vi "test Verify Timestamp Channels Created.vi"(8 "error in":errorcluster, 11 "TestCase in":refnum<class "Scripting.lvclass">) -> (0 "error out":errorcluster, 3 "TestCase out":refnum<class "Scripting.lvclass">)   [LabVIEW 2020, in "Scripting.lvclass"]
uses:
  Scripting.lvclass
  C:/dev/git/niveristand-custom-device-testing-tools/VeriStandScriptingTestCase/VeriStandScriptingTestCase.lvclass
  Shared/BIU Configuration.ctl
  Shared/Address.ctl
  Shared/Major Frame Definition.ctl
  Shared/Minor Frame Definition.ctl
  Shared/Acyclic Frame Definition.ctl
  Shared/Message Definition.ctl
  Shared/Message Type.ctl
  Shared/Terminal Endpoint.ctl
  Shared/Parameter Definition.ctl
  niveristand-custom-device-testing-tools/VeriStandScriptingTestCase/VeriStandScriptingTestCase.lvclass/VeriStandScriptingTestCase.ctl
  niveristand-custom-device-testing-tools/VeriStandScriptingTestCase/Read Target.vi
  Scripting/Constants.vi
  <vilib>/NI VeriStand/Custom Device Tools/Custom Device Utility Library/NI VeriStand - Search for All Items by GUID.vi
  NationalInstruments.VeriStand.SystemDefinitionAPI
  <vilib>/addons/_JKI Toolkits/VI Tester/TestCase.llb/TestCase.lvclass
  Scripting/AIM MIL-STD-1553 Scripting.lvlib
  <vilib>/NI VeriStand/Custom Device Tools/Custom Device Utility Library/Custom Device Utility Library.lvlib
  C:/Program Files (x86)/National Instruments/LabVIEW 2020/vi.lib/addons/_JKI Toolkits/VI Tester/TestCase.llb/TestCase.lvclass
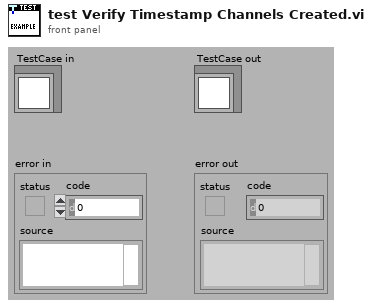
[diagram p1: front panel]
types:
  T1 = typedef "BIU Configuration.ctl" = cluster{"HW channel":u16, "terminal addresses":T2[], "terminal names":string[], "major frames":T3[], "minor frames":T4[], "acyclic frames":T5[], "messages":T6[], "minor frame period (us)":i32}
  T2 = typedef "Address.ctl" = u16
  T3 = typedef "Major Frame Definition.ctl" = cluster{"name":string, "minor frames":string[]}
  T4 = typedef "Minor Frame Definition.ctl" = cluster{"name":string, "messages":string[]}
  T5 = typedef "Acyclic Frame Definition.ctl" = cluster{"name":string, "messages":string[]}
  T6 = typedef "Message Definition.ctl" = cluster{"name":string, "message type":T7, "endpoint Tx":T8, "endpoint Rx":T8, "create timestamp channel":bool, "mode code":u16, "number of words":u16, "parameters":cluster{"name":string, "default value":dbl, "unit":string, "parameter definition":T9}[]}
  T7 = typedef "Message Type.ctl" = string
  T8 = typedef "Terminal Endpoint.ctl" = cluster{"terminal address":T2, "subaddress":T2}
  T9 = typedef "Parameter Definition.ctl" = cluster{"start index":i32, "size (bits)":i32, "encoding":enum16{"BNR", "BCD", "Discrete"}, "signed":bool, "multiplier":dbl, "offset":dbl}
  T10 = typedef "Custom Device API.lvlib/Custom Device Item Ref.ctl" = u64
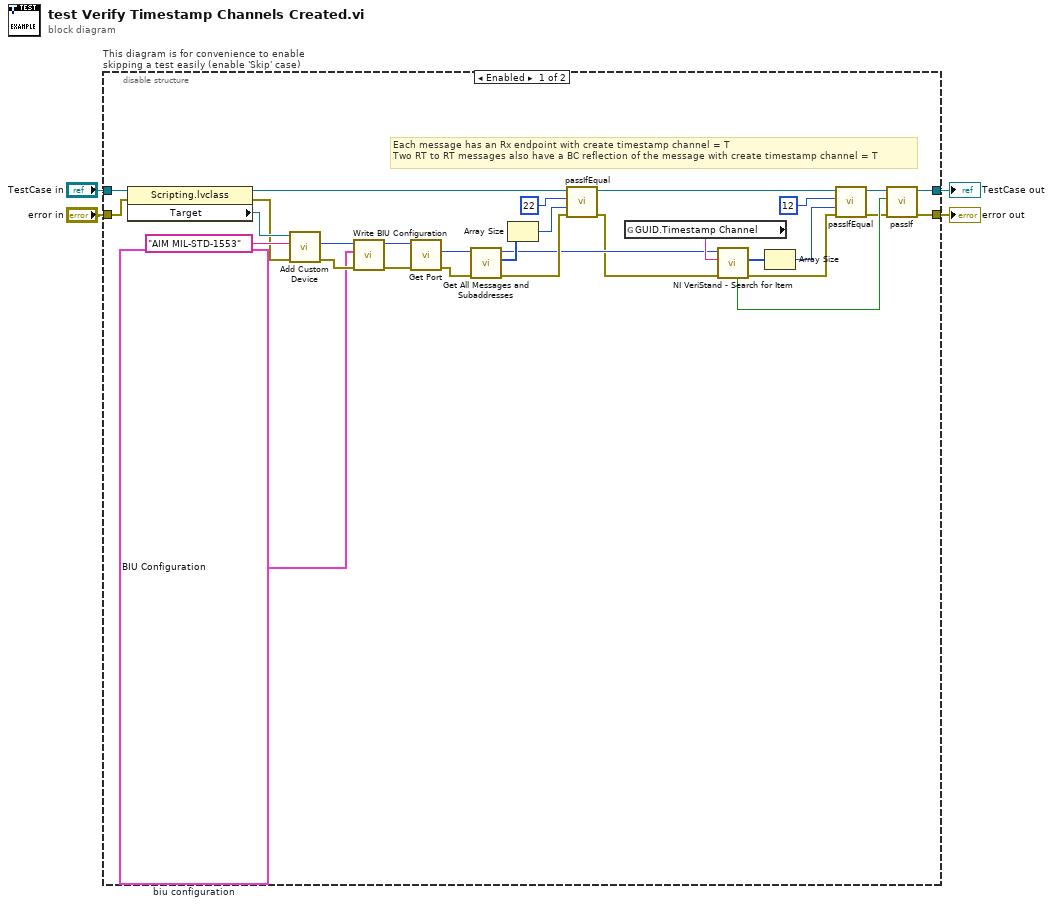
[diagram p0: block diagram]
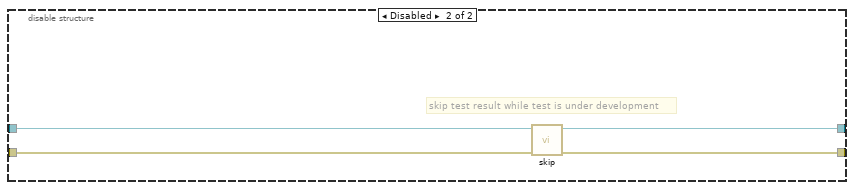
[diagram p2: hidden frame]
diagram:
  n1 = disable-structure "This diagram is for convenience to enable skipping a test easily (enable 'Skip' case)" shown="Enabled" {
    disable-tunnel: "TestCase in" -> [w33 w38]
    disable-tunnel: [w13 w36] -> w1
    disable-tunnel: [w14 w37] -> w3
    disable-tunnel: "error in" -> [w29 w35]
    frame Enabled {
      w9 = T1 {"HW channel"=0, "terminal addresses"=[0, 1, 15, 21, 31], "terminal names"=[], "major frames"=[], "minor frames"=[], "acyclic frames"=[{"name"="acyclicFrame ID56", "messages"=[]}], "messages"=[{"name"="BC to RT 1.2", "message type"="BC to RT", "endpoint Tx"={"terminal address"=0, "subaddress"=0}, "endpoint Rx"={"terminal address"=1, "subaddress"=2}, "create timestamp channel"=TRUE, "mode code"=0, "number of words"=3, "parameters"=[]}, {"name"="RT 31.15 to RT 21.21", "message type"="RT to RT", "endpoint Tx"={"terminal address"=15, "subaddress"=21}, "endpoint Rx"={"terminal address"=31, "subaddress"=21}, "create timestamp channel"=TRUE, "mode code"=0, "number of words"=11, "parameters"=[]}, {"name"="BC to RT 1.3", "message type"="BC to RT", "endpoint Tx"={"terminal address"=0, "subaddress"=0}, "endpoint Rx"={"terminal address"=1, "subaddress"=3}, "create timestamp channel"=TRUE, "mode code"=0, "number of words"=4, "parameters"=[]}, {"name"="RT 1.5 to BC", "message type"="RT to BC", "endpoint Tx"={"terminal address"=1, "subaddress"=5}, "endpoint Rx"={"terminal address"=0, "subaddress"=0}, "create timestamp channel"=TRUE, "mode code"=0, "number of words"=6, "parameters"=[]}, {"name"="RT 1.6 to BC", "message type"="RT to BC", "endpoint Tx"={"terminal address"=1, "subaddress"=6}, "endpoint Rx"={"terminal address"=0, "subaddress"=0}, "create timestamp channel"=TRUE, "mode code"=0, "number of words"=2, "parameters"=[]}, {"name"="RT 1.20 to RT 15.20", "message type"="RT to RT", "endpoint Tx"={"terminal address"=1, "subaddress"=20}, "endpoint Rx"={"terminal address"=15, "subaddress"=20}, "create timestamp channel"=TRUE, "mode code"=0, "number of words"=4, "parameters"=[]}, {"name"="MC 16", "message type"="MC", "endpoint Tx"={"terminal address"=1, "subaddress"=31}, "endpoint Rx"={"terminal address"=0, "subaddress"=0}, "create timestamp channel"=TRUE, "mode code"=16, "number of words"=1, "parameters"=[]}, {"name"="MC 17", "message type"="MC", "endpoint Tx"={"terminal address"=0, "subaddress"=0}, "endpoint Rx"={"terminal address"=1, "subaddress"=31}, "create timestamp channel"=TRUE, "mode code"=17, "number of words"=1, "parameters"=[]}, {"name"="BC to RT 31.28", "message type"="BC to RT", "endpoint Tx"={"terminal address"=0, "subaddress"=0}, "endpoint Rx"={"terminal address"=31, "subaddress"=28}, "create timestamp channel"=TRUE, "mode code"=0, "number of words"=6, "parameters"=[]}, {"name"="MC 1", "message type"="MC", "endpoint Tx"={"terminal address"=0, "subaddress"=0}, "endpoint Rx"={"terminal address"=31, "subaddress"=31}, "create timestamp channel"=TRUE, "mode code"=1, "number of words"=0, "parameters"=[]}], "minor frame period (us)"=0}  # biu configuration
      # "Each message has an Rx endpoint with create timestamp channel = T\nTwo RT to RT messages also have a BC reflection of the message with create timestamp channel = T"
      n2 = property class="Scripting.lvclass"(reference=w33, error in=w29) -> (reference out=w23:refnum<class "Scripting.lvclass">, error out=w28:errorcluster, "Target"=w32:refnum<k24>)
      n3 = call "Add Custom Device.vi"("error in"=w28, "custom device name"="AIM MIL-STD-1553" ("name"), "target"=w32) -> ("error out"=w30:errorcluster, "custom device"=w31:T10)  [unwired: 6 in, 1 out]
      n4 = call "Write BIU Configuration.vi"("error in"=w30, "biu configuration"=w9, "custom device"=w31) -> ("error out"=w7:errorcluster, "custom device out"=w8:T10)  [unwired: 7 in]
      n5 = call "Get Port.vi"("error in"=w7, "custom device ref"=w8) -> ("error out"=w6:errorcluster, "port"=w5:T10)  [unwired: 6 in, 2 out]
      n6 = call "Get All Messages and Subaddresses.vi"("error in"=w6, "port"=w5) -> ("error out"=w24:errorcluster, "messages and subaddresses"=w25:T10[], "port out"=w21:T10)  [unwired: 7 in]
      n7 = Array Size(array=w25) -> (size(s)=w27:i32)
      n8 = call-dynamic "passIfEqual.vi"("error in (no error)"=w24, "y"=w27, "x"=22 ("size(s)"), "TestCase in"=w23) -> ("error out"=w20:errorcluster, "TestCase out"=w19:refnum<class "Scripting.lvclass">)  [unwired: 6 in]
      n9 = global read "Constants.vi" "GUID.Timestamp Channel"() -> (w22:string)
      n10 = call-poly <vilib>:"NI VeriStand - Search for Item.vi"("error in"=w20, "Item GUID"=w22, "Section Ref in"=w21) -> ("error out"=w18:errorcluster, "Item Refs"=w12:T10[], "Found"=w17:bool)  [unwired: 5 in, 1 out]
      n11 = Array Size(array=w12) -> (size(s)=w11:i32)
      n12 = call-dynamic "passIfEqual.vi"("error in (no error)"=w18, "y"=w11, "x"=12 ("size(s)"), "TestCase in"=w19) -> ("error out"=w15:errorcluster, "TestCase out"=w16:refnum<class "Scripting.lvclass">)  [unwired: 6 in]
      n13 = call-dynamic "passIf.vi"("error in (no error)"=w15, "pass"=w17, "TestCase in"=w16) -> ("error out"=w14:errorcluster, "TestCase out"=w13:refnum<class "Scripting.lvclass">)  [unwired: 7 in]
    }
    frame Disabled {
      # "skip test result while test is under development"
      n14 = call <vilib>:"skip.vi"("error in (no error)"=w35, "TestCase in"=w38) -> ("error out"=w37:errorcluster, "TestCase out"=w36:refnum<class "Scripting.lvclass">)  [unwired: 8 in]
    }
  }
  "error out" <- w3
  "TestCase out" <- w1
